vi "Unsubscribe.vi"(8 "error in (no error)":errorcluster, 9 "Subscriber Enqueuer":refnum<class "Message Enqueuer.lvclass">, 10 "Topic":string, 11 "Broadcaster in":refnum<class "BroadcastBroker.lvclass">) -> (0 "error out":errorcluster, 3 "Broadcaster out":refnum<class "BroadcastBroker.lvclass">)   [LabVIEW 2019, in "BroadcastBroker.lvclass"]
uses:
  BroadcastBroker.lvclass
  <vilib>/ActorFramework/Message Enqueuer/Message Enqueuer.lvclass
  BroadcastBroker.lvclass/BroadcastBroker.ctl
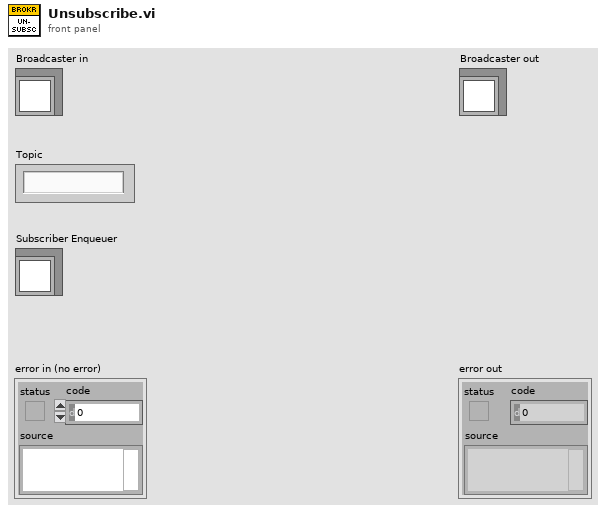
[diagram p1: front panel]
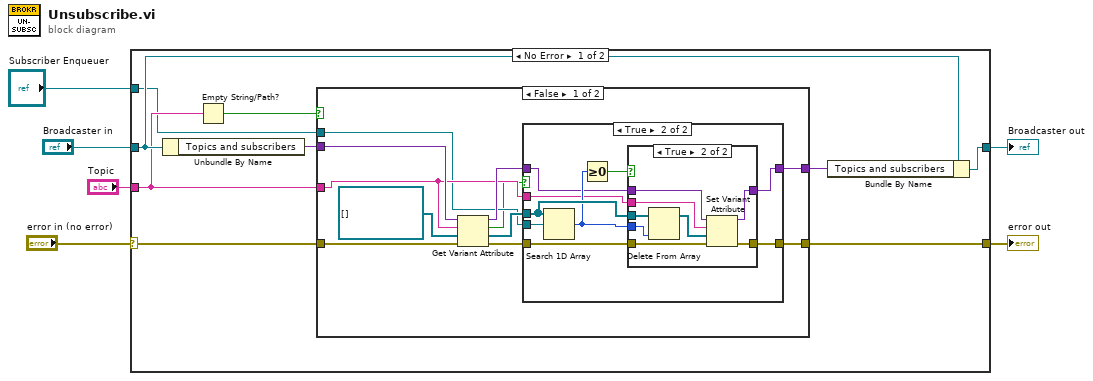
[diagram p0: block diagram]
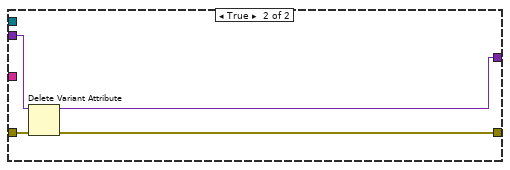
[diagram p4: hidden frame]
diagram:
  n1 = case shown="No Error" "error in (no error)" {
    selector: "error in (no error)" -> [w13 w53]
    tunnel: [w10 w53] -> w5
    tunnel: [w12 w52] -> w3
    tunnel: "Broadcaster in" -> [w15 w52]
    tunnel: "Topic" -> [w9 _]
    tunnel: "Subscriber Enqueuer" -> [w8 _]
    frame No Error {
      n2 = Unbundle By Name(w15) -> ("Topics and subscribers"=w14:variant)
      n3 = Empty String/Path?(string/path=w9) -> (empty?=w7:bool)
      n4 = case shown="False" w7 {
        tunnel: w14 -> [w26 w51]
        tunnel: w13 -> [w25 w50]
        tunnel: [w22 w48] -> w11
        tunnel: [w21 w49] -> w10
        tunnel: w9 -> [w19 _]
        tunnel: w8 -> [w18 _]
        frame False {
          n5 = Get Variant Attribute(Variant=w26, name=w19, default value (empty Variant)=refnum<class "Message Enqueuer.lvclass">[] [], error in=w25) -> (duplicate Variant=w23:variant, found=w16:bool, value=w20:refnum<class "Message Enqueuer.lvclass">[], error out=w24:errorcluster)
          n6 = case shown="True" w16 {
            tunnel: w24 -> [w27 w31]
            tunnel: w23 -> [w28 w33]
            tunnel: [w28 w30] -> w22
            tunnel: [w27 w29] -> w21
            tunnel: w20 -> [_ w36]
            tunnel: w19 -> [_ w32]
            tunnel: w18 -> [_ w34]
            frame False {
            }
            frame True {
              n7 = Search 1D Array(1D array=w36, element=w34) -> (index of element=w35:i32)  [unwired: 1 in]
              n8 = Greater Or Equal To 0?(x=w35) -> (x >= 0?=w37:bool)
              n9 = case shown="True" w37 {
                tunnel: w36 -> [_ w47]
                tunnel: w35 -> [_ w46]
                tunnel: w33 -> [w39 w45]
                tunnel: w32 -> [_ w44]
                tunnel: w31 -> [w38 w42]
                tunnel: [w39 w41] -> w30
                tunnel: [w38 w40] -> w29
                frame False {
                }
                frame True {
                  n10 = Delete From Array(array=w47, index=w46) -> (array with subset deleted=w43:refnum<class "Message Enqueuer.lvclass">[])  [unwired: 1 in, 1 out]
                  n11 = Set Variant Attribute(Variant=w45, name=w44, value=w43, error in=w42) -> (Variant out=w41:variant, error out=w40:errorcluster)  [unwired: 1 out]
                }
              }
            }
          }
        }
        frame True {
          n12 = Delete Variant Attribute(4:w50, 7:w51) -> (0:w49:errorcluster, 3:w48:variant)  [unwired: 1 in, 1 out]
        }
      }
      n13 = Bundle By Name(cluster=w15, "Topics and subscribers"=w11) -> (w12:refnum<class "BroadcastBroker.lvclass">)
    }
    frame Error {
    }
  }
  "error out" <- w5
  "Broadcaster out" <- w3
